vi "Blink - TCP Connection.vi"() -> ()   [LabVIEW 2011, in "LVH-LINX.lvlib"]
doc: "Read one or more analog values from a LINX device using the LINX serial interface."
uses:
  vi.lib/LabVIEW Hacker/LINX/LVH-LINX.lvlib
  vi.lib/LabVIEW Hacker/LINX/Private/Device/Type Defs/TCP Config.ctl
  vi.lib/LabVIEW Hacker/LINX/Private/Type Defs/Interface.ctl
  vi.lib/LabVIEW Hacker/LINX/Private/Device/Device.lvlib
panel:
  in  "TCP Configuration":T1
  out "LED Value":bool
  in  "Digital Output Channel":u8=13
  out "Loop Rate (Hz)":u32
  in  "Stop Button":bool
  # "LINX Device Settings"
  # "LED Value"
  # "Blink (TCP Interface)\n\nThis example demonstrates how to blink an LED on a LINX device connected to \nthe host computer using TCP.\n\nInstructions\n1. Select the IP Address  and Port associated with the LINX Device.\n2. Select the Digital Pin connected to the LED.\n3. Click the Run Arrow."
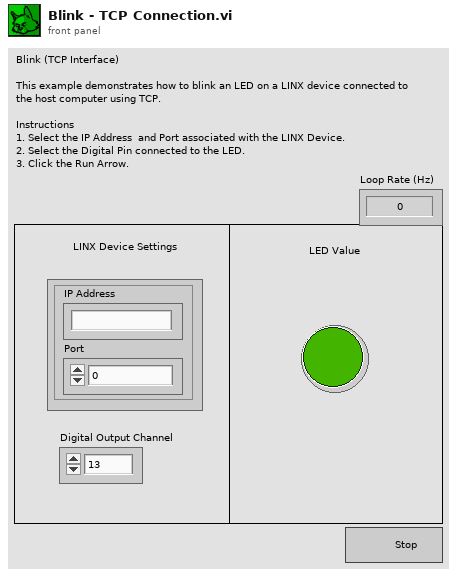
[diagram p1: front panel]
types:
  T1 = typedef "LVH-LINX.lvlib/Device.lvlib/TCP Config.ctl" = cluster{"IP Address":string, "Port":u16}
  T2 = typedef "LVH-LINX.lvlib/Interface.ctl" = enum16{"Serial", "TCP"}
  T3 = typedef "LVH-LINX.lvlib/LINX Ref.ctl" = cluster{"Platform":T4, "Interface":T2, "LINX Device Config":T5}
  T4 = typedef "LVH-LINX.lvlib/Platform.ctl" = enum16{"LINX", "myRIO"}
  T5 = typedef "LVH-LINX.lvlib/Device.lvlib/LINX Device Config.ctl" = cluster{"Interface":T2, "COM Port":refnum<visa-resource-name>, "TCP Configuration":T1, "Device Family":T6, "Device ID":u8, "Device Name":string, "TCP Ref":refnum<k5>}
  T6 = typedef "LVH-LINX.lvlib/Device Family.ctl" = enum8{"National Instruments", "Digilent", "Arduino"}
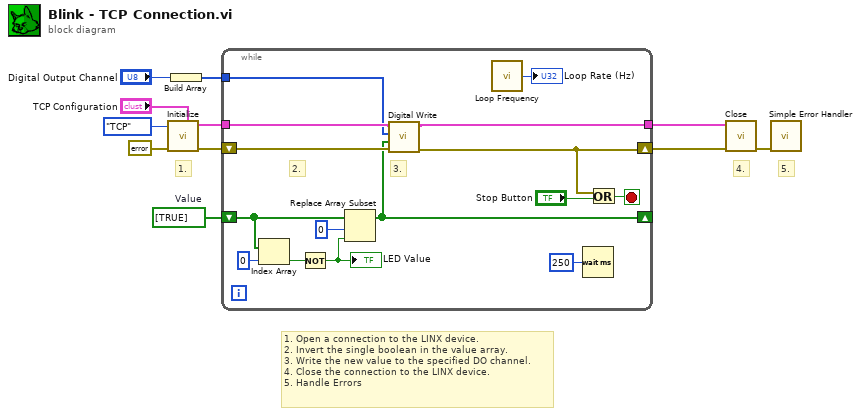
[diagram p0: block diagram]
diagram:
  w3 = bool[] [TRUE]  # Value
  # "1. Open a connection to the LINX device.\n2. Invert the single boolean in the value array.\n3. Write the new value to the specified DO channel.\n4. Close the connection to the LINX device.\n5. Handle Errors"
  # "5."
  # "4."
  # "1."
  n1 = call "Initialize.vi"("TCP Configuration"="TCP Configuration", "Error In"=errorcluster {"status"=FALSE, "code"=0, "source"=""}, "Interface"=Interface."TCP") -> ("Error Out"=w10:errorcluster, "LINX Ref"=w11:T3)  [unwired: 6 in, 1 out]
  n2 = Build Array("Digital Output Channel") -> (w4:u8[])
  n3 = while {
    tunnel: w11 -> [w23]
    tunnel: [w22] -> w9
    shift-right: [w20] -> w8
    shift-left: w10 -> [w21]
    tunnel: w4 -> [w19]
    shift-right: [w13] -> _
    shift-left: w3 -> [w18]
    stop <- w26 stop-if-true
    # "2."
    # "3."
    n4 = Index Array(array=w18, index=0) -> (element=w16:bool)
    n5 = Not(x=w16) -> (.not. x?=w15:bool)
    "LED Value" <- w15
    n6 = Replace Array Subset(array=w18, new element=w15, index=0) -> (w13:bool[])
    n7 = call "Digital Write.vi"("Error In"=w21, "Values"=w13, "Channels"=w19, "LINX Resource"=w23) -> ("Error Out"=w20:errorcluster, "LINX Resource"=w22:T3)  [unwired: 6 in]
    n8 = call "Loop Frequency.vi"() -> ("Loop Rate (Hz)"=→"Loop Rate (Hz)":u32)
    n9 = Wait (ms)(milliseconds to wait=u32 250) -> ()  [unwired: 1 out]
    n10 = Or(x=w20, y="Stop Button") -> (x .or. y?=w26:bool)
  }
  n11 = call "Close.vi"("Error In"=w8, "LINX Resource"=w9) -> ("Error Out"=w7:errorcluster)  [unwired: 8 in, 1 out]
  n12 = call <vilib>:"Simple Error Handler.vi"("error in (no error)"=w7) -> ()  [unwired: 4 in, 5 out]
